vi "TagBus_Create Key Strings from Controls.vi"(10 "Array":refnum<vi>[](array[refnum]), 11 "Process Name":string) -> (3 "Key Array":string[](array[string]))   [LabVIEW 2015, in "TagBus.lvclass"]
uses:
  TagBus.lvclass
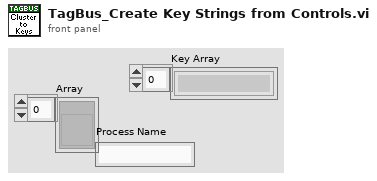
[diagram p1: front panel]
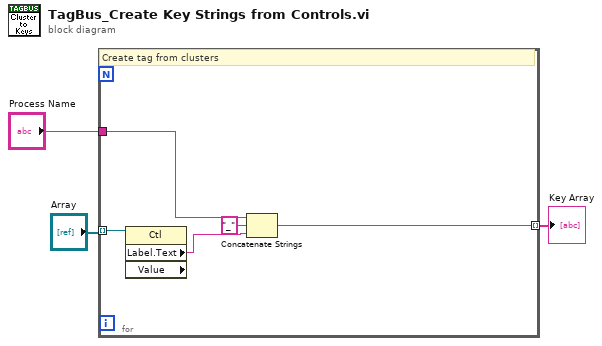
[diagram p0: block diagram]
diagram:
  n1 = for {
    tunnel: "Array" -> [w8] mode=indexing
    tunnel: "Process Name" -> [w6]
    tunnel: [w4] -> w1 mode=indexing
    # "Create tag from clusters"
    n2 = property class="Ctl" props=["Label", "Text", "Value"](reference=w8) -> ("Label.Text"=w7:string)  [unwired: 1 in, 3 out]
    n3 = Concatenate Strings(w6, "_" ("string"), w7) -> (w4:string)
  }
  "Key Array" <- w1
